vi "624FastTalonReadEncoderData.vi"(10 "Reset?":bool, 11 "CAN Talon SRX Ref":T1={"DeviceStatus"={"status"=FALSE, "code"=0, "source"=""}, "Type"=enum."PWM", "PWM"={"PWM Channel"=enum."PWM 1", "DeadBand"={"Name"="", "maxPositivePwm"=0, "minPositivePwm"=0, "centerPwm"=0, "maxNegativePwm"=0, "minNegativePwm"=0, "angularRange"=0}}, "CAN"={"Device Number"=0, "Control Mode"=enum."Percent VBus", "Semaphore"=refnum, "Max Vout"=12.0, "TalonSRX Control Mode"=enum."Percent VBus"}, "Invert"=FALSE}) -> (2 "Sensor RPM":dbl, 3 "Sensor Position":dbl)   [LabVIEW 2015]
uses:
  <vilib>/Rock Robotics/WPI/MotorControl/WPI_MotorControlDeviceRef.ctl
  <vilib>/Rock Robotics/WPI/MotorControl/WPI_MotorControlType.ctl
  <vilib>/Rock Robotics/SystemInterfaces/DIO/FPGA_DIOPWMChannel.ctl
  <vilib>/Rock Robotics/WPI/PWM/WPI_PWMDeadband.ctl
  <vilib>/Rock Robotics/WPI/CAN/Jaguar/SubVIs/WPI_CANJaguar_ControlMode.ctl
  <vilib>/Rock Robotics/WPI/CAN/TalonSRX/WPI_CANTalonSRX_APIControlMode.ctl
  <vilib>/Rock Robotics/WPI/CAN/TalonSRX/WPI_CANTalonSRX_MessageIDs.ctl
panel:
  out "Vel Div 4?":bool
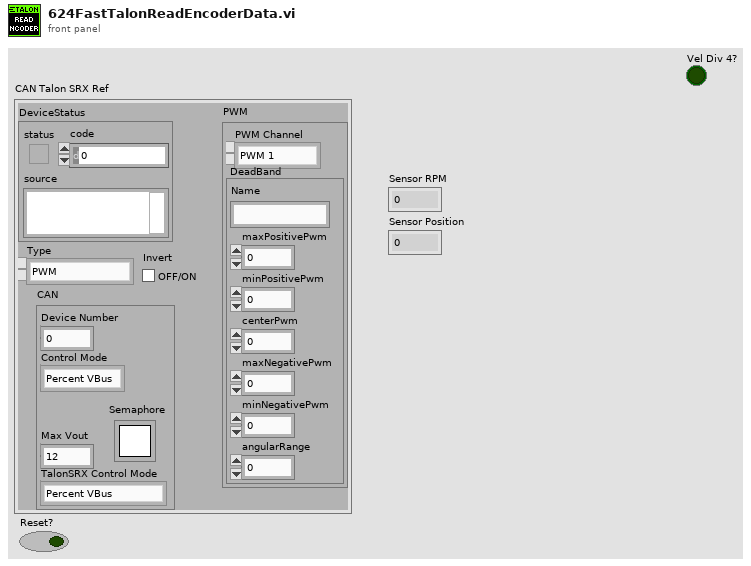
[diagram p1: front panel]
types:
  T1 = typedef "WPI_MotorControlDeviceRef.ctl" = cluster{"DeviceStatus":errorcluster, "Type":T2, "PWM":cluster{"PWM Channel":T3, "DeadBand":T4}, "CAN":cluster{"Device Number":u8, "Control Mode":T5, "Semaphore":T6, "Max Vout":dbl, "TalonSRX Control Mode":T7}, "Invert":bool}
  T2 = typedef "WPI_MotorControlType.ctl" = enum16{"PWM", "CAN", "CANTalonSRX"}
  T3 = typedef "FPGA_DIOPWMChannel.ctl" = enum8{"PWM 0", "PWM 1", "PWM 2", "PWM 3", "PWM 4", "PWM 5", "PWM 6", "PWM 7", "PWM 8", "PWM 9", "PWM MXP 0", "PWM MXP 1", "PWM MXP 2", "PWM MXP 3", "PWM MXP 4", "PWM MXP 5", "PWM MXP 6", "PWM MXP 7", "PWM MXP 8", "PWM MXP 9", "Invalid"}
  T4 = typedef "WPI_PWMDeadband.ctl" = cluster{"Name":string, "maxPositivePwm":i32, "minPositivePwm":i32, "centerPwm":i32, "maxNegativePwm":i32, "minNegativePwm":i32, "angularRange":u16}
  T5 = typedef "WPI_CANJaguar_ControlMode.ctl" = enum8{"Percent VBus", "Current", "Speed", "Position", "Voltage"}
  T6 = typedef "Semaphore RefNum" = refnum<k1>
  T7 = typedef "WPI_CANTalonSRX_APIControlMode.ctl" = enum8{"Percent VBus", "Speed", "Position", "Slave", "Unchanged / Invalid", "Voltage Compensation", "Current", "Motion Profile"}
  T8 = typedef "WPI_CANTalonSRX_MessageIDs.ctl" = u32
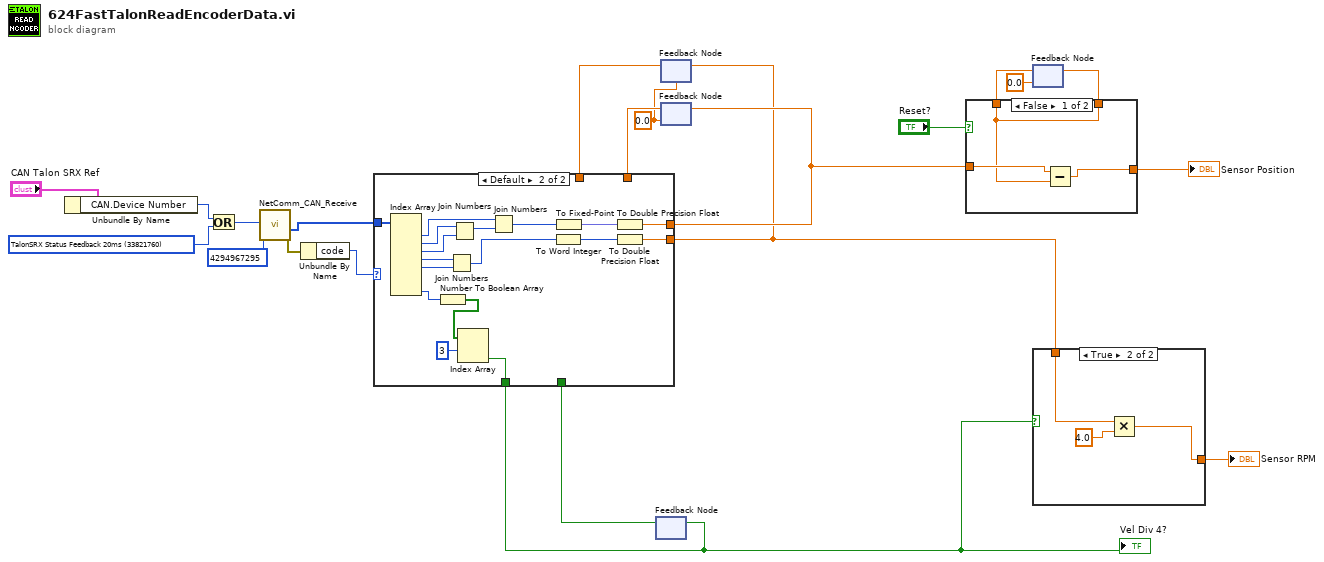
[diagram p0: block diagram]
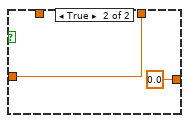
[diagram p3: hidden frame]
diagram:
  w5 = 0.0
  w18 = T8 33821760 items=["TalonSRX Control General 10ms"=33816576, "TalonSRX Control Rates Slow"=33816640, "TalonSRX Control ClearFlags Slow"=33816704, "TalonSRX Status General 10ms"=33821696, "TalonSRX Status Feedback 20ms"=33821760, "TalonSRX Status Enc 100ms"=33821824, "TalonSRX Status AinTempVbat 100ms"=33821888, "TalonSRX Status Startup Once"=33821952, "TalonSRX Status Debug"=33822080, "TalonSRX Config SetGainsSlot0 A"=33823808, "TalonSRX Config SetGainsSlot0 B"=33823872, "TalonSRX Config SetGainsSlot1 A"=33823936, "TalonSRX Config SetGainsSlot1 B"=33824000, "TalonSRX Config SetSoftLimits"=33824064, "TalonSRX Config WebControl"=33824128, "TalonSRX Param Request"=33822720, "TalonSRX Param Response"=33822784, "TalonSRX Param Set"=33822848]
  n1 = Unbundle By Name("CAN Talon SRX Ref") -> ("CAN.Device Number"=w19:u8)
  n2 = Or(x=w19, y=w18) -> (x .or. y?=w17:T8)
  n3 = call <vilib>:"NetComm_CAN_Receive.vi"("Message ID Mask"=u32 4294967295, "Message ID"=w17) -> ("error out"=w16:errorcluster, "Data"=w20:u8[])  [unwired: 1 in, 7 out]
  n4 = Unbundle By Name(w16) -> ("code"=w15:i32)
  n5 = feedback #1() -> (w4:bool)  [unwired: 1 in]
  n6 = feedback #2(w5) -> (w12:dbl)
  n7 = feedback #3(w5) -> (w13:dbl)
  n8 = case shown="Default" w15 {
    tunnel: w20 -> [_ w30]
    tunnel: [w24 w29] -> w10
    tunnel: [w23 w28] -> w2
    tunnel: w13 -> [w24 _]
    tunnel: w12 -> [w23 _]
    tunnel: [w22 w25] -> w3
    tunnel: w4 -> [w22 _]
    frame -44087 {
    }
    frame Default {
      n9 = Index Array(array=w30) -> (element #1=w39:u8, element #2=w41:u8, element #3=w38:u8, element #4=w37:u8, element #5=w36:u8, element #8=w34:u8)  [unwired: 8 in, 2 out]
      n10 = Number To Boolean Array(number=w34) -> (Boolean array=w27:bool[])
      n11 = Join Numbers(hi=w37, lo=w36) -> ((hi.lo)=w35:u16)
      n12 = Join Numbers(hi=w41, lo=w38) -> ((hi.lo)=w40:u16)
      n13 = Index Array(array=w27, index #1=3 ("index")) -> (element #2=w25:bool)  [unwired: 1 in, 1 out]
      n14 = Join Numbers(hi=w39, lo=w40) -> ((hi.lo)=w32:u32)
      n15 = To Word Integer(number=w35) -> (16bit integer=w33:i16)
      n16 = To Fixed-Point(number=w32) -> (fixed-point=w31:fxp<+/-,24,24>)  [unwired: 1 in]
      n17 = To Double Precision Float(number=w31) -> (double precision float=w29:dbl)
      n18 = To Double Precision Float(number=w33) -> (double precision float=w28:dbl)
    }
  }
  "Vel Div 4?" <- w3
  n19 = feedback-in #1(w3) -> ()
  n20 = feedback-in #2(w2) -> ()
  n21 = feedback-in #3(w10) -> ()
  n22 = feedback #4(0.0) -> (w8:dbl)
  n23 = case shown="False" "Reset?" {
    tunnel: w10 -> [w44 w46]
    tunnel: [w43 w46] -> w9
    tunnel: w8 -> [w43 _]
    tunnel: [w42 0.0] -> w7
    frame False {
      n24 = Subtract(x=w44, y=w43) -> (x-y=w42:dbl)
    }
    frame True {
    }
  }
  "Sensor Position" <- w7
  n25 = feedback-in #4(w9) -> ()
  n26 = case shown="True" w3 {
    tunnel: w2 -> [w47 w50]
    tunnel: [w47 w48] -> w1
    frame False {
    }
    frame True {
      n27 = Multiply(x=w50, y=4.0) -> (x*y=w48:dbl)
    }
  }
  "Sensor RPM" <- w1
